vi "Add Node.vi"(7 "Parent Path":string, 8 "Attributes":map{string, string}(c390), 9 "Data":string, 10 "New Node Name":string, 11 "Tree Map In":T1) -> (0 "Path Invalid":bool, 3 "Tree Map Out":T1, 5 "New Node Path":string)   [LabVIEW 2019, in "Tree Map.lvlib"]
doc: "Add a node to the Tree Map. Data asociated with this node can be optionally specified.\n\n<b>NOTE</b> Be careful not to use XML special characters for the data or name of the node if you intend to flatten and unflatten from XML. This can cause error in XML functions.\n\n<b>Author:</b> Piotr Kruczkowski <PrimaryKey>\n<b>License:</b> NewBSD\n\nCopyright (c) 2019, National Instruments\nAll rights reserved.\n\nRedistribution and use in source and binary forms, with or without\nmodification, are permitted provided that the following conditions are met:\n1. Redistributions of source code must retain the above copyright\n notice, this list of conditions and the following disclaimer.\n2. Redistributions in binary form must reproduce the above copyright\n notice, this list of conditions and the following disclaimer in the\n documentation and/or other materials provided with the distribution.\n3. Neither the name of National Instruments nor the\n names of its contributors may be used to endorse or promote products\n derived from this software without specific prior written permission.\n\nTHIS SOFTWARE IS PROVIDED BY National Instruments ''AS IS'' AND ANY\nEXPRESS OR IMPLIED WARRANTIES, INCLUDING, BUT NOT LIMITED TO, THE IMPLIED\nWARRANTIES OF MERCHANTABILITY AND FITNESS FOR A PARTICULAR PURPOSE ARE\nDISCLAIMED. IN NO EVENT SHALL National Instruments BE LIABLE FOR ANY\nDIRECT, INDIRECT, INCIDENTAL, SPECIAL, EXEMPLARY, OR CONSEQUENTIAL DAMAGES\n(INCLUDING, BUT NOT LIMITED TO, PROCUREMENT OF SUBSTITUTE GOODS OR SERVICES;\nLOSS OF USE, DATA, OR PROFITS; OR BUSINESS INTERRUPTION) HOWEVER CAUSED AND\nON ANY THEORY OF LIABILITY, WHETHER IN CONTRACT, STRICT LIABILITY, OR TORT\n(INCLUDING NEGLIGENCE OR OTHERWISE) ARISING IN ANY WAY OUT OF THE USE OF THIS\nSOFTWARE, EVEN IF ADVISED OF THE POSSIBILITY OF SUCH DAMAGE."
uses:
  Tree Map.lvlib
  Tree Map Data.ctl
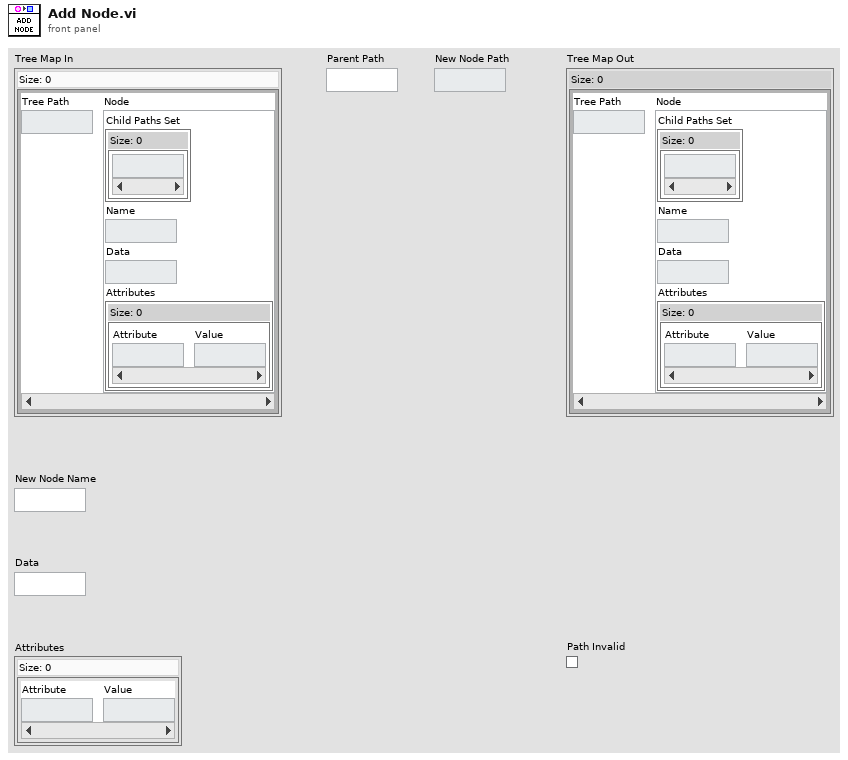
[diagram p1: front panel]
types:
  T1 = typedef "Tree Map.lvlib/Tree Map Data.ctl" = map{string, cluster{"Child Paths Set":set{string}, "Name":string, "Data":string, "Attributes":map{string, string}}}
  T2 = cluster{"Child Paths Set":set{string}, "Name":string, "Data":string, "Attributes":map{string, string}}
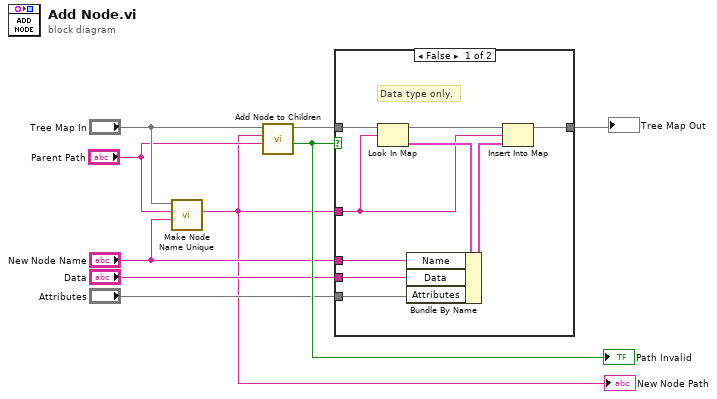
[diagram p0: block diagram]
diagram:
  n1 = call "Make Node Name Unique.vi"("New Node Name"="New Node Name", "Parent Path"="Parent Path", "Tree Map In"="Tree Map In") -> ("Node Path"=w1:string)  [unwired: 8 in]
  "New Node Path" <- w1
  n2 = call "Add Node to Children.vi"("Parent Path"="Parent Path", "Node Path"=w1, "Tree Map In"="Tree Map In") -> ("Path Invalid"=w9:bool, "Tree Map Out"=w5:T1)  [unwired: 7 in]
  "Path Invalid" <- w9
  n3 = case shown="False" w9 {
    tunnel: w5 -> [w16 w18]
    tunnel: w1 -> [w13 _]
    tunnel: [w17 w18] -> w7
    tunnel: "Data" -> [w12 _]
    tunnel: "Attributes" -> [w11 _]
    tunnel: "New Node Name" -> [w10 _]
    frame False {
      # "Data type only."
      n4 = Look In Map(map=w16, key=w13) -> (value=w15:T2)  [unwired: 1 in, 1 out]
      n5 = Bundle By Name(cluster=w15, "Name"=w10, "Data"=w12, "Attributes"=w11) -> (w14:T2)
      n6 = Insert Into Map(map in=w16, key=w13, value=w14) -> (map out=w17:T1)  [unwired: 2 out]
    }
    frame True {
    }
  }
  "Tree Map Out" <- w7
